vi "PatternMatchIkW.vi"(0 "SerRead":string, 2 "StreamingBytesPerFrame":i16=140) -> (3 "CorrectedSubstring":string, 4 "lengthCorr":i32, 5 "firstFrame":string, 6 "foundMatch":bool)   [LabVIEW 2017]
panel:
  out "index of element":i32
  out "U16Data":u16[](array[numeric])
  out "iter":i32
  out "NframesIn":i32
  out "Nframesout":i32
  out "match I":string
  out "offset past match kW":i32
  out "after subStr kW":string
  out "match kW":string
  out "LengthIn":i32
  out "offset past match":i32
  out "after subStr I":string
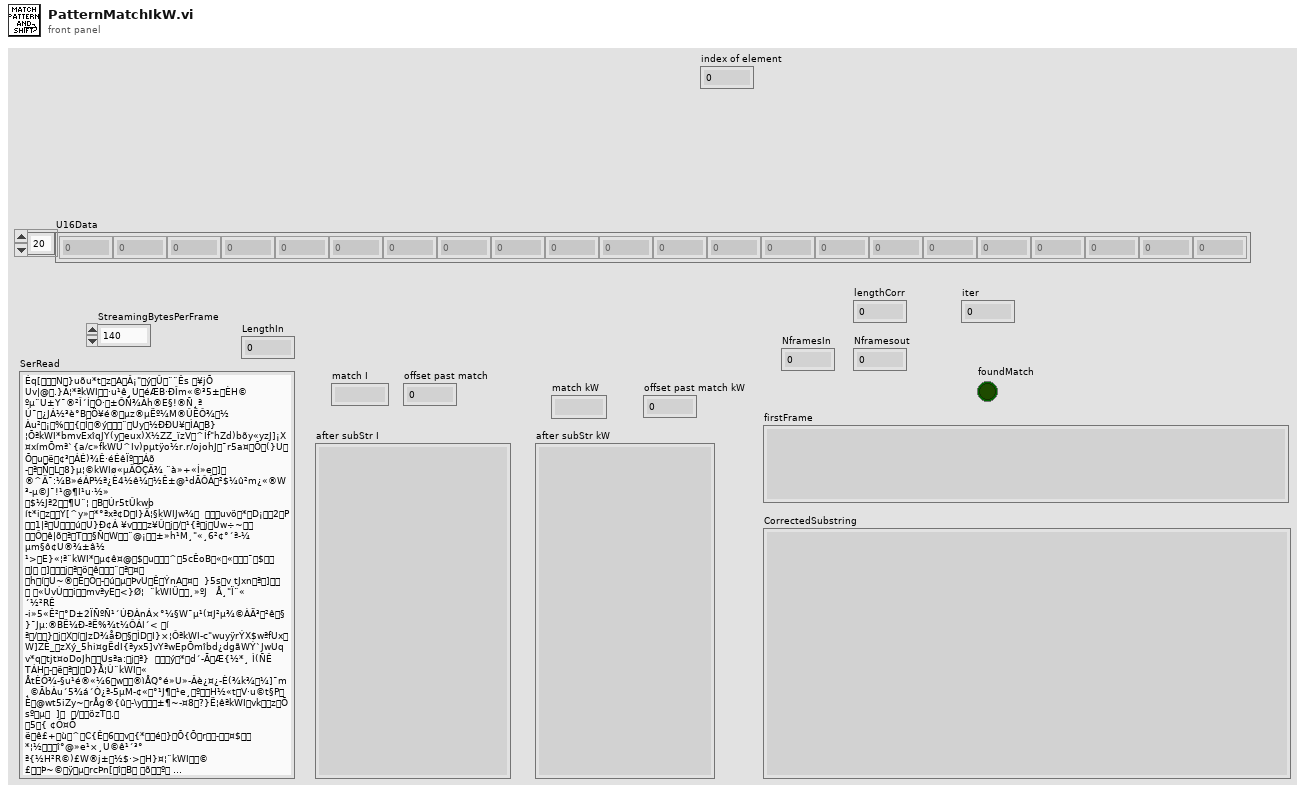
[diagram p1: front panel]
types:
  T1 = enum16{"big-endian, network order", "native, host order", "little-endian"}
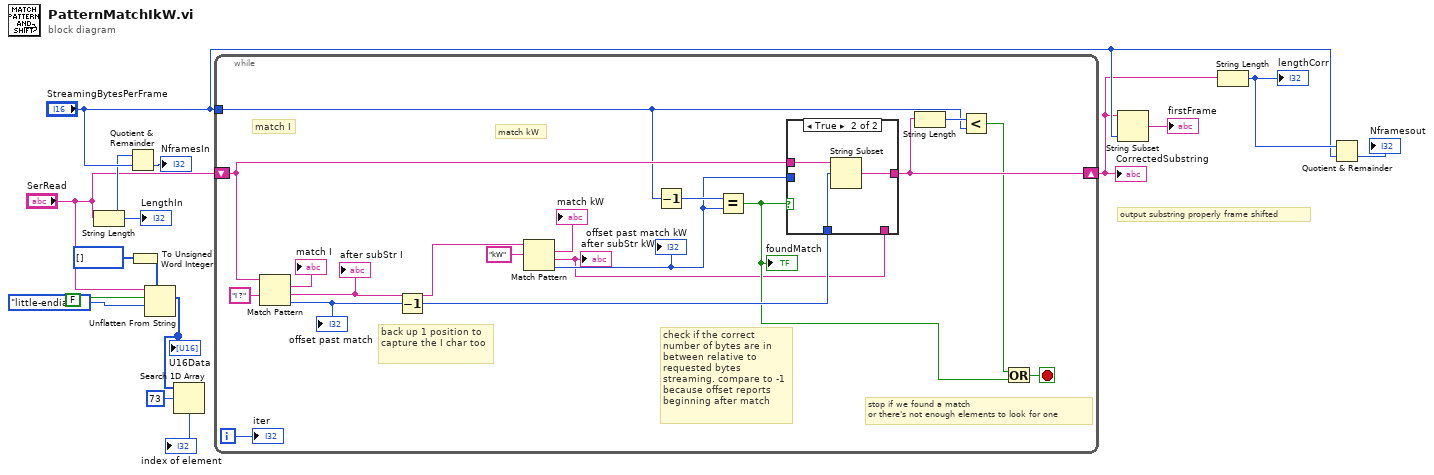
[diagram p0: block diagram]
diagram:
  # "output substring properly frame shifted"
  n1 = String Length(string="SerRead") -> (length=w11:i32)
  "LengthIn" <- w11
  n2 = Quotient & Remainder(x=w11, y="StreamingBytesPerFrame") -> (floor(x/y)=→"NframesIn":i32)  [unwired: 1 out]
  n3 = To Unsigned Word Integer(number=i16[] []) -> (unsigned 16bit integer=w4:u16[])
  n4 = Unflatten From String(type=w4, binary string="SerRead", data includes array or string size? (T)=FALSE, byte order (0:big-endian, network order)=T1."little-endian") -> (value=w3:u16[])  [unwired: 1 in, 2 out]
  "U16Data" <- w3
  n5 = Search 1D Array(1D array=w3, element=u16 73) -> (index of element=→"index of element":i32)  [unwired: 1 in]
  n6 = while {
    tunnel: "StreamingBytesPerFrame" -> [w21]
    shift-right: [w23] -> w9
    shift-left: "SerRead" -> [w28]
    i -> [w24]
    stop <- w18 stop-if-true
    # "stop if we found a match\nor there's not enough elements to look for one"
    # "back up 1 position to capture the I char too"
    # "check if the correct number of bytes are in between relative to requested bytes streaming. compare to -1 because offset reports beginning after match"
    # "match kW"
    # "match I"
    n7 = Match Pattern(string=w28, regular expression="I ?") -> (match substring=→"match I":string, after substring=w27:string, offset past match=w30:i32)  [unwired: 1 in, 1 out]
    "after subStr I" <- w27
    "offset past match" <- w30
    n8 = Decrement(x=w30) -> (x-1=w29:i32)
    n9 = Match Pattern(string=w27, regular expression="kW") -> (match substring=→"match kW":string, after substring=w16:string, offset past match=w17:i32)  [unwired: 1 in, 1 out]
    "after subStr kW" <- w16
    "offset past match kW" <- w17
    n10 = Decrement(x=w21) -> (x-1=w26:i16)
    n11 = Equal?(x=w26, y=w17) -> (x = y?=w19:bool)
    "foundMatch" <- w19
    n12 = case shown="True" w19 {
      tunnel: w29 -> [_ w37]
      tunnel: w28 -> [_ w36]
      tunnel: [w34 w35] -> w23
      tunnel: w17 -> [_ _]
      tunnel: w16 -> [w34 _]
      frame False {
      }
      frame True {
        n13 = String Subset(string=w36, offset (0)=w37) -> (substring=w35:string)  [unwired: 1 in]
      }
    }
    n14 = String Length(string=w23) -> (length=w22:i32)
    n15 = Less?(x=w22, y=w21) -> (x < y?=w20:bool)
    n16 = Or(x=w20, y=w19) -> (x .or. y?=w18:bool)
    "iter" <- w24
  }
  "CorrectedSubstring" <- w9
  n17 = String Subset(string=w9, length (rest)="StreamingBytesPerFrame") -> (substring=→"firstFrame":string)  [unwired: 1 in]
  n18 = String Length(string=w9) -> (length=w14:i32)
  "lengthCorr" <- w14
  n19 = Quotient & Remainder(x=w14, y="StreamingBytesPerFrame") -> (floor(x/y)=→"Nframesout":i32)  [unwired: 1 out]
